vi "Aurora Create Resources (Dual Port).vi"(10 "RX CLIP Resources":T5, 11 "TX CLIP Resources":T6) -> (2 "aurora rx dual reference":T1, 3 "aurora tx dual reference":T3)   [LabVIEW 2019]
doc: "Creates an AXI4-Stream Address Space Collection with the selected <b>CLIP Resources</b> at the appropriate offsets.\n\n<B>Input Parameters</B>\n\n<B>RX CLIP Resources</B> specifies the CLIP resources to use for the RX portion of AXI4-Stream.\n\n<B>TX CLIP Resources</B> specifies the CLIP resources to use for the TX portion of AXI4-Stream.\n\n<B>Output Parameters</B>\n\n<B>RX niInstr AXI4-Stream Reader FXP64x4 v1 FPGA out</B> passes a reference to the newly-created RX AXI4-Stream Reader to the next VI.\n\n<B>TX niInstr AXI4-Stream Writer FXP64x4 v1 FPGA out</B> passes a reference to the newly-created TX AXI4-Stream Writer to the next VI."
uses:
  Aurora TX Dual Reference.ctl
  AXI4-Stream Writer FXP64x4 Resources.ctl
  Aurora RX Dual Reference.ctl
  AXI4-Stream Reader FXP64x4 Resources.ctl
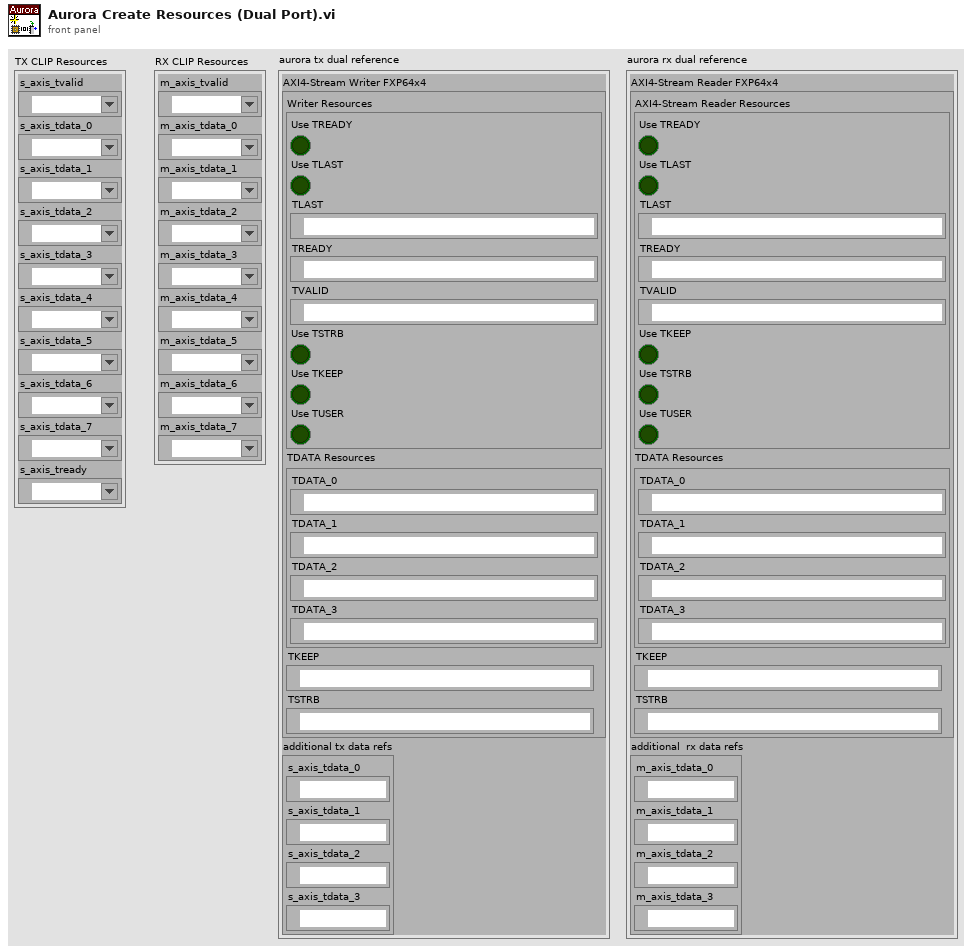
[diagram p1: front panel]
types:
  T1 = typedef "Aurora RX Dual Reference.ctl" = cluster{"AXI4-Stream Reader FXP64x4":T2, "additional  rx data refs":cluster{"m_axis_tdata_0":refnum<k21>, "m_axis_tdata_1":refnum<k21>, "m_axis_tdata_2":refnum<k21>, "m_axis_tdata_3":refnum<k21>}}
  T2 = typedef "AXI4-Stream Reader FXP64x4 Resources.ctl" = cluster{"AXI4-Stream Reader Resources":cluster{"Use TREADY":bool, "Use TLAST":bool, "TLAST":refnum<k21>, "TREADY":refnum<k21>, "TVALID":refnum<k21>, "Use TKEEP":bool, "Use TSTRB":bool, "Use TUSER":bool}, "TDATA Resources":cluster{"TDATA_0":refnum<k21>, "TDATA_1":refnum<k21>, "TDATA_2":refnum<k21>, "TDATA_3":refnum<k21>}, "TKEEP":refnum<k21>, "TSTRB":refnum<k21>}
  T3 = typedef "Aurora TX Dual Reference.ctl" = cluster{"AXI4-Stream Writer FXP64x4":T4, "additional tx data refs":cluster{"s_axis_tdata_0":refnum<k21>, "s_axis_tdata_1":refnum<k21>, "s_axis_tdata_2":refnum<k21>, "s_axis_tdata_3":refnum<k21>}}
  T4 = typedef "AXI4-Stream Writer FXP64x4 Resources.ctl" = cluster{"Writer Resources":cluster{"Use TREADY":bool, "Use TLAST":bool, "TLAST":refnum<k21>, "TREADY":refnum<k21>, "TVALID":refnum<k21>, "Use TSTRB":bool, "Use TKEEP":bool, "Use TUSER":bool}, "TDATA Resources":cluster{"TDATA_0":refnum<k21>, "TDATA_1":refnum<k21>, "TDATA_2":refnum<k21>, "TDATA_3":refnum<k21>}, "TKEEP":refnum<k21>, "TSTRB":refnum<k21>}
  T5 = cluster{"m_axis_tvalid":refnum<k21>, "m_axis_tdata_0":refnum<k21>, "m_axis_tdata_1":refnum<k21>, "m_axis_tdata_2":refnum<k21>, "m_axis_tdata_3":refnum<k21>, "m_axis_tdata_4":refnum<k21>, "m_axis_tdata_5":refnum<k21>, "m_axis_tdata_6":refnum<k21>, "m_axis_tdata_7":refnum<k21>}
  T6 = cluster{"s_axis_tvalid":refnum<k21>, "s_axis_tdata_0":refnum<k21>, "s_axis_tdata_1":refnum<k21>, "s_axis_tdata_2":refnum<k21>, "s_axis_tdata_3":refnum<k21>, "s_axis_tdata_4":refnum<k21>, "s_axis_tdata_5":refnum<k21>, "s_axis_tdata_6":refnum<k21>, "s_axis_tdata_7":refnum<k21>, "s_axis_tready":refnum<k21>}
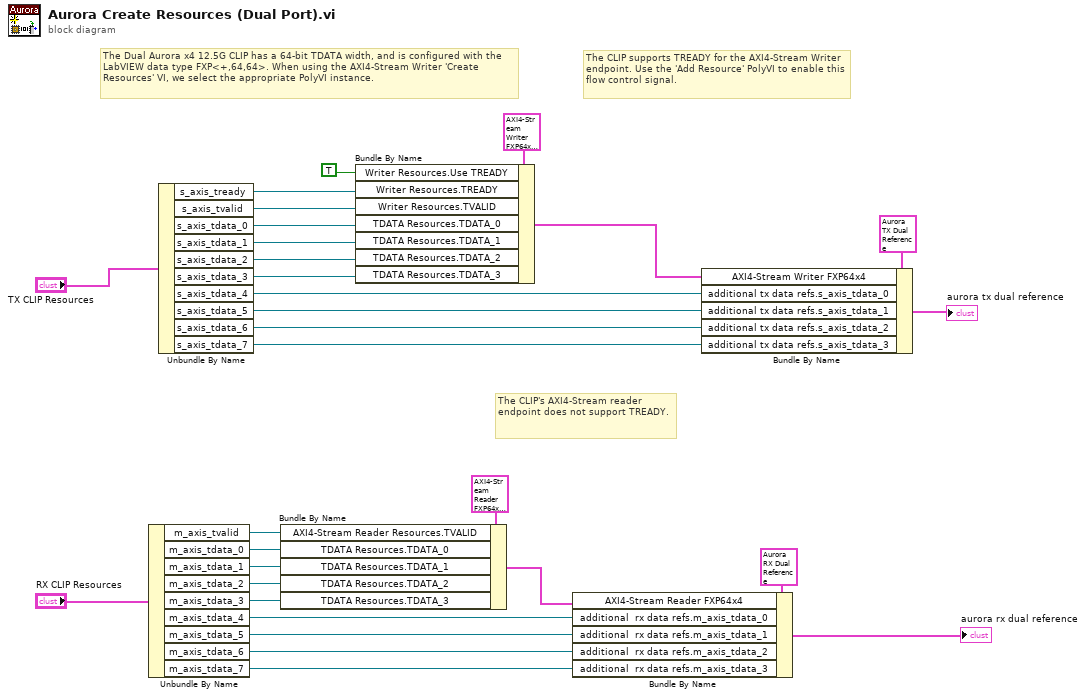
[diagram p0: block diagram]
diagram:
  # "The CLIP's AXI4-Stream reader endpoint does not support TREADY."
  # "The CLIP supports TREADY for the AXI4-Stream Writer endpoint. Use the 'Add Resource' PolyVI to enable this flow control signal."
  # "The Dual Aurora x4 12.5G CLIP has a 64-bit TDATA width, and is configured with the LabVIEW data type FXP<+,64,64>. When using the AXI4-Stream Writer 'Create Resources' VI, we select the appropriate PolyVI instance."
  n1 = Unbundle By Name("RX CLIP Resources") -> ("m_axis_tvalid"=w10:refnum<k21>, "m_axis_tdata_0"=w9:refnum<k21>, "m_axis_tdata_1"=w8:refnum<k21>, "m_axis_tdata_2"=w7:refnum<k21>, "m_axis_tdata_3"=w6:refnum<k21>, "m_axis_tdata_4"=w4:refnum<k21>, "m_axis_tdata_5"=w3:refnum<k21>, "m_axis_tdata_6"=w2:refnum<k21>, "m_axis_tdata_7"=w1:refnum<k21>)
  n2 = Unbundle By Name("TX CLIP Resources") -> ("s_axis_tready"=w24:refnum<k21>, "s_axis_tvalid"=w23:refnum<k21>, "s_axis_tdata_0"=w22:refnum<k21>, "s_axis_tdata_1"=w21:refnum<k21>, "s_axis_tdata_2"=w20:refnum<k21>, "s_axis_tdata_3"=w19:refnum<k21>, "s_axis_tdata_4"=w15:refnum<k21>, "s_axis_tdata_5"=w14:refnum<k21>, "s_axis_tdata_6"=w13:refnum<k21>, "s_axis_tdata_7"=w12:refnum<k21>)
  n3 = Bundle By Name(cluster=T2 {"AXI4-Stream Reader Resources"={"Use TREADY"=FALSE, "Use TLAST"=FALSE, "TLAST"="", "TREADY"="", "TVALID"="", "Use TKEEP"=FALSE, "Use TSTRB"=FALSE, "Use TUSER"=FALSE}, "TDATA Resources"={"TDATA_0"="", "TDATA_1"="", "TDATA_2"="", "TDATA_3"=""}, "TKEEP"="", "TSTRB"=""} ("AXI4-Stream Reader FXP64x4"), "AXI4-Stream Reader Resources.TVALID"=w10, "TDATA Resources.TDATA_0"=w9, "TDATA Resources.TDATA_1"=w8, "TDATA Resources.TDATA_2"=w7, "TDATA Resources.TDATA_3"=w6) -> (w5:T2)
  n4 = Bundle By Name(cluster=T4 {"Writer Resources"={"Use TREADY"=FALSE, "Use TLAST"=FALSE, "TLAST"="", "TREADY"="", "TVALID"="", "Use TSTRB"=FALSE, "Use TKEEP"=FALSE, "Use TUSER"=FALSE}, "TDATA Resources"={"TDATA_0"="", "TDATA_1"="", "TDATA_2"="", "TDATA_3"=""}, "TKEEP"="", "TSTRB"=""} ("AXI4-Stream Writer FXP64x4"), "Writer Resources.Use TREADY"=TRUE, "Writer Resources.TREADY"=w24, "Writer Resources.TVALID"=w23, "TDATA Resources.TDATA_0"=w22, "TDATA Resources.TDATA_1"=w21, "TDATA Resources.TDATA_2"=w20, "TDATA Resources.TDATA_3"=w19) -> (w16:T4)
  n5 = Bundle By Name(cluster=T1 {"AXI4-Stream Reader FXP64x4"={"AXI4-Stream Reader Resources"={"Use TREADY"=FALSE, "Use TLAST"=FALSE, "TLAST"="", "TREADY"="", "TVALID"="", "Use TKEEP"=FALSE, "Use TSTRB"=FALSE, "Use TUSER"=FALSE}, "TDATA Resources"={"TDATA_0"="", "TDATA_1"="", "TDATA_2"="", "TDATA_3"=""}, "TKEEP"="", "TSTRB"=""}, "additional  rx data refs"={"m_axis_tdata_0"="", "m_axis_tdata_1"="", "m_axis_tdata_2"="", "m_axis_tdata_3"=""}} ("aurora rx dual reference"), "AXI4-Stream Reader FXP64x4"=w5, "additional  rx data refs.m_axis_tdata_0"=w4, "additional  rx data refs.m_axis_tdata_1"=w3, "additional  rx data refs.m_axis_tdata_2"=w2, "additional  rx data refs.m_axis_tdata_3"=w1) -> (→"aurora rx dual reference":T1)
  n6 = Bundle By Name(cluster=T3 {"AXI4-Stream Writer FXP64x4"={"Writer Resources"={"Use TREADY"=FALSE, "Use TLAST"=FALSE, "TLAST"="", "TREADY"="", "TVALID"="", "Use TSTRB"=FALSE, "Use TKEEP"=FALSE, "Use TUSER"=FALSE}, "TDATA Resources"={"TDATA_0"="", "TDATA_1"="", "TDATA_2"="", "TDATA_3"=""}, "TKEEP"="", "TSTRB"=""}, "additional tx data refs"={"s_axis_tdata_0"="", "s_axis_tdata_1"="", "s_axis_tdata_2"="", "s_axis_tdata_3"=""}} ("aurora tx dual reference"), "AXI4-Stream Writer FXP64x4"=w16, "additional tx data refs.s_axis_tdata_0"=w15, "additional tx data refs.s_axis_tdata_1"=w14, "additional tx data refs.s_axis_tdata_2"=w13, "additional tx data refs.s_axis_tdata_3"=w12) -> (→"aurora tx dual reference":T3)
